vi "Shutdown Daemon.vi"(8 "error in":errorcluster, 11 "network slave in":refnum<class "Network Slave.lvclass">) -> (0 "error out":errorcluster)   [LabVIEW 2021, in "Network Slave.lvclass"]
doc: "This provides an interface for the slave to shut down its protocol daemon."
uses:
  Network Slave.lvclass
  Network Slave.lvclass/Network Slave.ctl
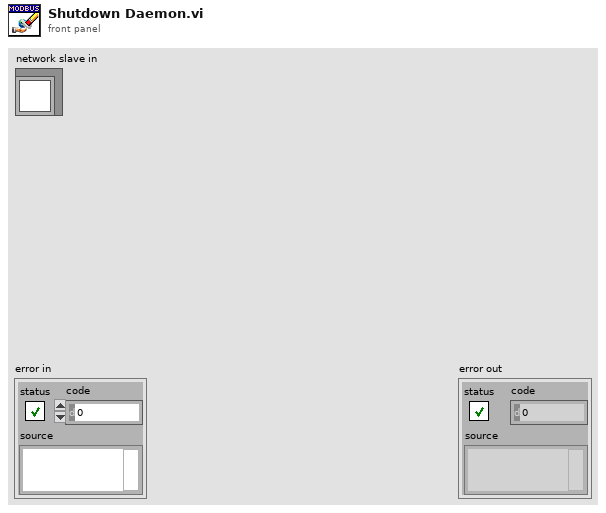
[diagram p1: front panel]
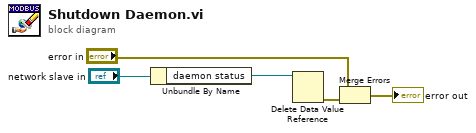
[diagram p0: block diagram]
diagram:
  n1 = Unbundle By Name("network slave in") -> ("daemon status"=w5:refnum<data-value>)
  n2 = Delete Data Value Reference(data value reference=w5) -> (error out=w4:errorcluster)  [unwired: 1 in, 1 out]
  n3 = Merge Errors("error in", w4) -> (→"error out":errorcluster)
